vi "InitializePowerSupply.vi"(9 "Serial Configuration":T1={"Parity(0:none)"=0, "Baud Rate (9600)"=9600, "Data Bits(8)"=8, "Flow Control(None)"=0, " Stop Bits(1.0)"=10} {"Stop Bits(1.0)" items=["1.0"=10, "1.5"=15, "2.0"=20]; "Flow Control(None)" items=["None", "XON/XOFF", "RTS/CTS", "XON/XOFF & RTS/CTS", "DTR/DSR", "XON/XOFF & DTR/DSR"]; "Data Bits(8)" items=["7"=7, "8"=8]; "Baud Rate (9600)" items=["2400"=2400, "4800"=4800, "9600"=9600, "19200"=19200, "38400"=38400]; "Parity(0:none)" items=["None", "Odd", "Even", "Mark", "Space"]}, 10 "Manual Range(0.00)":dbl format="%.2f", 11 "VISA resource name":refnum<visa-resource-name>) -> (2 "error out":errorcluster, 3 "VISA resource name out":refnum<visa-resource-name>)   [LabVIEW 2009]
uses:
  <instrlib>/BK Precision 91xx Series/BK Precision 91xx Series.lvlib
panel:
  in  "Unit(V)":u16(ring) items=["V", "mV", "kV", "A", "mA"]
  in  "Function(0:Voltage)":u16(ring) items=["Voltage", "Current"]
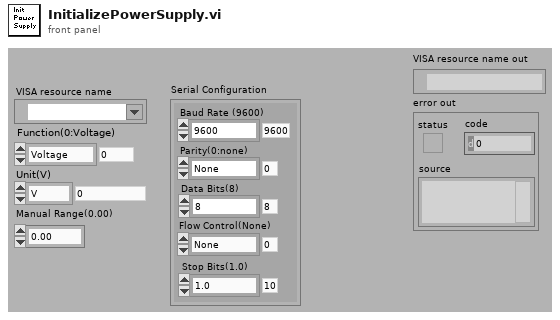
[diagram p1: front panel]
types:
  T1 = cluster{"Parity(0:none)":u16, "Baud Rate (9600)":u16, "Data Bits(8)":u16, "Flow Control(None)":u16, " Stop Bits(1.0)":u16}
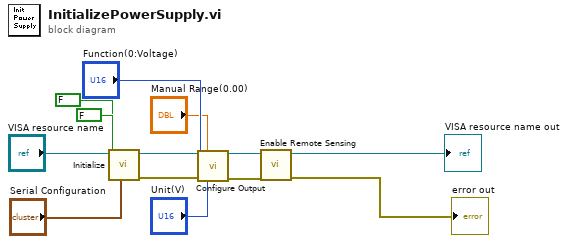
[diagram p0: block diagram]
diagram:
  n1 = call <instrlib>:"Initialize.vi"("Serial Configuration"="Serial Configuration", "Reset (True)"=FALSE, "ID Query (True)"=FALSE, "VISA resource name"="VISA resource name") -> ("error out"=w10:errorcluster, "VISA resource name out"=w12:refnum<visa-resource-name>)  [unwired: 6 in]
  n2 = call <instrlib>:"Configure Output.vi"("VISA resource name"=w12, "Manual Range(0.00)"="Manual Range(0.00)", "Function(0:Voltage)"="Function(0:Voltage)", "error in (no error)"=w10, "Unit(V)"="Unit(V)") -> ("VISA resource name out"=w9:refnum<visa-resource-name>, "error out"=w8:errorcluster)  [unwired: 9 in]
  n3 = call <instrlib>:"Enable Remote Sensing.vi"("error in (no error)"=w8, "VISA resource name"=w9) -> ("error out"=→"error out":errorcluster, "VISA resource name out"=→"VISA resource name out":refnum<visa-resource-name>)  [unwired: 8 in]
